vi "Define Global Constants.vi"   [LabVIEW 2014]
uses:
  Global Constants.vi
panel:
  # "INSTRUCTIONS:\n\nTo add a constant, create a string constant with your constant's name. Then copy the \"Read Config File\" vi and hook your constant into the \"key\" input. Then hook the \"value\" into your Global Constant. Make sure that you have defined your constant in the _config.ini file or it will not read your constant.\n\nSee the example constant if you are confused."
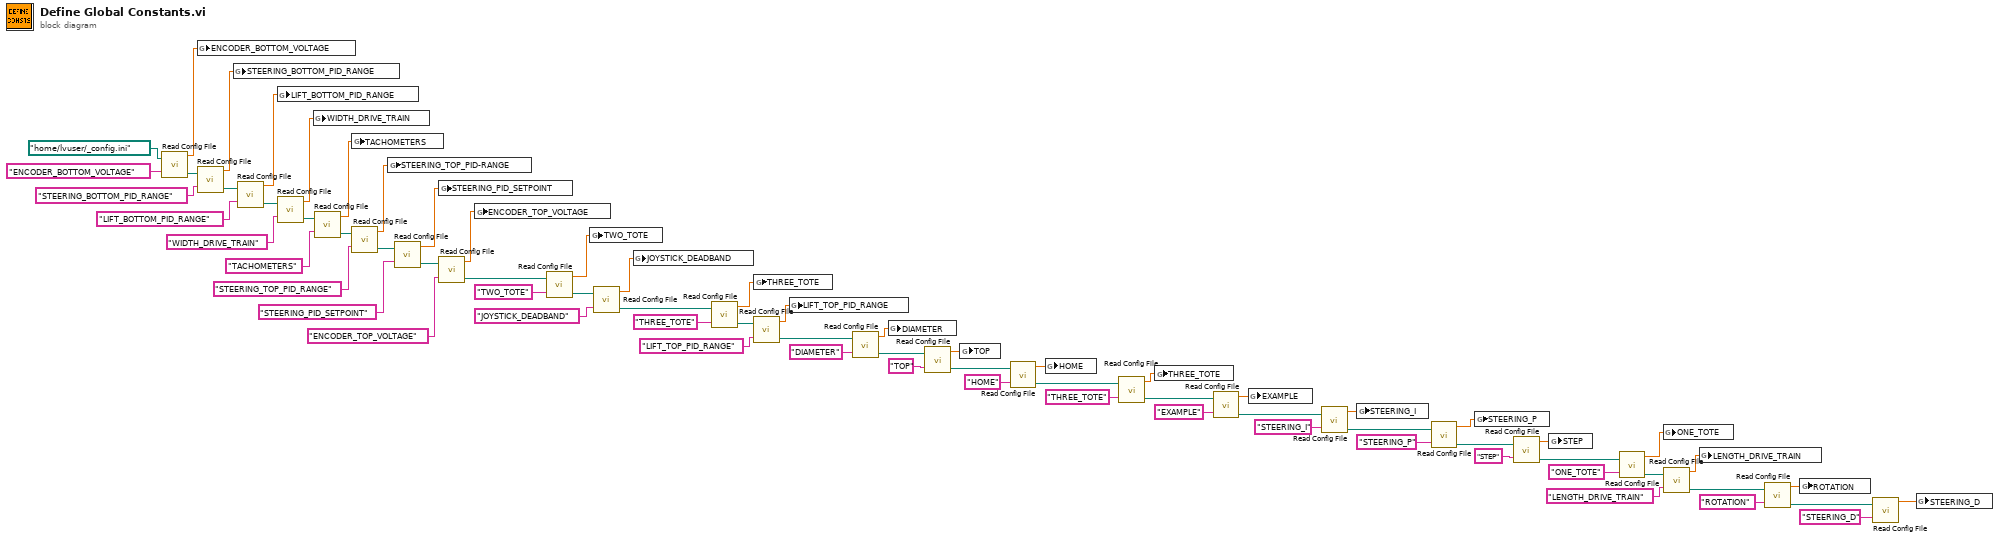
[diagram p0: block diagram]
diagram:
  n1 = call "Read Config File.vi"("file path"=path "/home/lvuser/_config.ini" ("configuration file path"), "key"="ENCODER_BOTTOM_VOLTAGE") -> ("value"=w40:dbl, "file path"=w23:path)  [unwired: 1 out]
  n2 = global write "Global Constants.vi" "ENCODER_BOTTOM_VOLTAGE"(w40) -> ()
  n3 = call "Read Config File.vi"("file path"=w23, "key"="STEERING_BOTTOM_PID_RANGE") -> ("value"=w39:dbl, "file path"=w22:path)  [unwired: 1 out]
  n4 = global write "Global Constants.vi" "STEERING_BOTTOM_PID_RANGE"(w39) -> ()
  n5 = call "Read Config File.vi"("file path"=w22, "key"="LIFT_BOTTOM_PID_RANGE") -> ("value"=w47:dbl, "file path"=w21:path)  [unwired: 1 out]
  n6 = global write "Global Constants.vi" "LIFT_BOTTOM_PID_RANGE"(w47) -> ()
  n7 = call "Read Config File.vi"("file path"=w21, "key"="WIDTH_DRIVE_TRAIN") -> ("value"=w41:dbl, "file path"=w20:path)  [unwired: 1 out]
  n8 = global write "Global Constants.vi" "WIDTH_DRIVE_TRAIN"(w41) -> ()
  n9 = call "Read Config File.vi"("file path"=w20, "key"="TACHOMETERS") -> ("value"=w35:dbl, "file path"=w19:path)  [unwired: 1 out]
  n10 = global write "Global Constants.vi" "TACHOMETERS"(w35) -> ()
  n11 = call "Read Config File.vi"("file path"=w19, "key"="STEERING_TOP_PID_RANGE") -> ("value"=w52:dbl, "file path"=w18:path)  [unwired: 1 out]
  n12 = global write "Global Constants.vi" "STEERING_TOP_PID-RANGE"(w52) -> ()
  n13 = call "Read Config File.vi"("file path"=w18, "key"="STEERING_PID_SETPOINT") -> ("value"=w46:dbl, "file path"=w17:path)  [unwired: 1 out]
  n14 = global write "Global Constants.vi" "STEERING_PID_SETPOINT"(w46) -> ()
  n15 = call "Read Config File.vi"("file path"=w17, "key"="ENCODER_TOP_VOLTAGE") -> ("value"=w45:dbl, "file path"=w16:path)  [unwired: 1 out]
  n16 = global write "Global Constants.vi" "ENCODER_TOP_VOLTAGE"(w45) -> ()
  n17 = call "Read Config File.vi"("file path"=w16, "key"="TWO_TOTE") -> ("value"=w51:dbl, "file path"=w15:path)  [unwired: 1 out]
  n18 = global write "Global Constants.vi" "TWO_TOTE"(w51) -> ()
  n19 = call "Read Config File.vi"("file path"=w15, "key"="JOYSTICK_DEADBAND") -> ("value"=w44:dbl, "file path"=w12:path)  [unwired: 1 out]
  n20 = global write "Global Constants.vi" "JOYSTICK_DEADBAND"(w44) -> ()
  n21 = call "Read Config File.vi"("file path"=w12, "key"="THREE_TOTE") -> ("value"=w50:dbl, "file path"=w14:path)  [unwired: 1 out]
  n22 = global write "Global Constants.vi" "THREE_TOTE"(w50) -> ()
  n23 = call "Read Config File.vi"("file path"=w14, "key"="LIFT_TOP_PID_RANGE") -> ("value"=w43:dbl, "file path"=w13:path)  [unwired: 1 out]
  n24 = global write "Global Constants.vi" "LIFT_TOP_PID_RANGE"(w43) -> ()
  n25 = call "Read Config File.vi"("file path"=w13, "key"="DIAMETER") -> ("value"=w31:dbl, "file path"=w11:path)  [unwired: 1 out]
  n26 = global write "Global Constants.vi" "DIAMETER"(w31) -> ()
  n27 = call "Read Config File.vi"("file path"=w11, "key"="TOP") -> ("value"=w28:dbl, "file path"=w10:path)  [unwired: 1 out]
  n28 = global write "Global Constants.vi" "TOP"(w28) -> ()
  n29 = call "Read Config File.vi"("file path"=w10, "key"="HOME") -> ("value"=w27:dbl, "file path"=w9:path)  [unwired: 1 out]
  n30 = global write "Global Constants.vi" "HOME"(w27) -> ()
  n31 = call "Read Config File.vi"("file path"=w9, "key"="THREE_TOTE") -> ("value"=w37:dbl, "file path"=w8:path)  [unwired: 1 out]
  n32 = global write "Global Constants.vi" "THREE_TOTE"(w37) -> ()
  n33 = call "Read Config File.vi"("file path"=w8, "key"="EXAMPLE") -> ("value"=w72:dbl, "file path"=w7:path)  [unwired: 1 out]
  n34 = global write "Global Constants.vi" "EXAMPLE"(w72) -> ()
  n35 = call "Read Config File.vi"("file path"=w7, "key"="STEERING_I") -> ("value"=w67:dbl, "file path"=w6:path)  [unwired: 1 out]
  n36 = global write "Global Constants.vi" "STEERING_I"(w67) -> ()
  n37 = call "Read Config File.vi"("file path"=w6, "key"="STEERING_P") -> ("value"=w69:dbl, "file path"=w5:path)  [unwired: 1 out]
  n38 = global write "Global Constants.vi" "STEERING_P"(w69) -> ()
  n39 = call "Read Config File.vi"("file path"=w5, "key"="STEP") -> ("value"=w38:dbl, "file path"=w4:path)  [unwired: 1 out]
  n40 = global write "Global Constants.vi" "STEP"(w38) -> ()
  n41 = call "Read Config File.vi"("file path"=w4, "key"="ONE_TOTE") -> ("value"=w48:dbl, "file path"=w3:path)  [unwired: 1 out]
  n42 = global write "Global Constants.vi" "ONE_TOTE"(w48) -> ()
  n43 = call "Read Config File.vi"("file path"=w3, "key"="LENGTH_DRIVE_TRAIN") -> ("value"=w42:dbl, "file path"=w2:path)  [unwired: 1 out]
  n44 = global write "Global Constants.vi" "LENGTH_DRIVE_TRAIN"(w42) -> ()
  n45 = call "Read Config File.vi"("file path"=w2, "key"="ROTATION") -> ("value"=w33:dbl, "file path"=w1:path)  [unwired: 1 out]
  n46 = global write "Global Constants.vi" "ROTATION"(w33) -> ()
  n47 = call "Read Config File.vi"("file path"=w1, "key"="STEERING_D") -> ("value"=w49:dbl)  [unwired: 2 out]
  n48 = global write "Global Constants.vi" "STEERING_D"(w49) -> ()
